vi "Get Path.vi"(8 "error in (no error)":errorcluster) -> (0 "error out (no error)":errorcluster, 2 "Library Path":path)   [LabVIEW 2020, in "lvzstd.lvlib"]
uses:
  lvzstd.lvlib
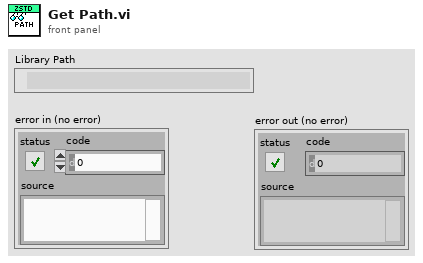
[diagram p1: front panel]
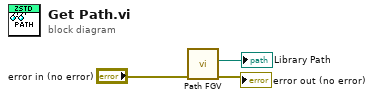
[diagram p0: block diagram]
diagram:
  n1 = call "Path FGV.vi"("error in (no error)"="error in (no error)") -> ("error out (no error)"=→"error out (no error)":errorcluster, "Library Path"=→"Library Path":path)  [unwired: 9 in]
